vi "Save As Tiff.vi"(7 "typ":i32, 8 "error in (no error)":errorcluster, 9 "position":i32, 10 "palette":string, 11 "path":string) -> (0 "error out":errorcluster, 1 "function return":u32, 2 "palette out":string, 3 "path out":string)   [LabVIEW 2014, in "atmcd32d.lvlib"]
doc: "unsigned int WINAPI SaveAsTiff(char * path, char * palette, int position, int typ);"
uses:
  atmcd32d.lvlib
  atmcd32d.dll
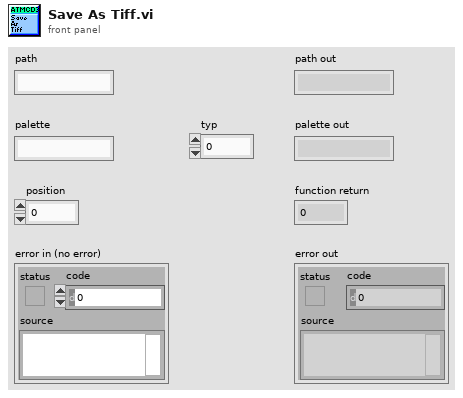
[diagram p1: front panel]
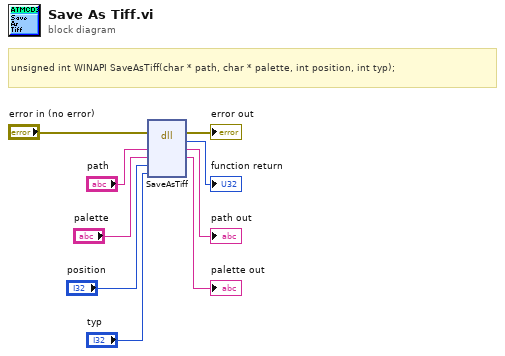
[diagram p0: block diagram]
diagram:
  # "unsigned int WINAPI SaveAsTiff(char * path, char * palette, int position, int typ);"
  n1 = dll-call lib="C:/Users/Bakir/Documents/Lambda2-Testing/lib/Andorlib/atmcd32d.*" fn="SaveAsTiff"(error in="error in (no error)", "path"="path", "palette"="palette", "position"="position", "typ"="typ") -> (error out=→"error out":errorcluster, →"function return":u32, "path"=→"path out":string, "palette"=→"palette out":string)  [unwired: 4 in, 1 out]
